vi "wash reactor.vi"(1 "channel":i8=1, 2 "Switch to position (A/B)":enum16{"A", "B"}(ring)) -> ()   [LabVIEW 2023]
panel:
  out "channel":string
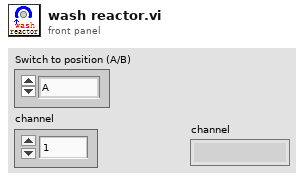
[diagram p1: front panel]
types:
  T1 = enum16{"Initialize", "Absolute Position", "Relative Pickup", "Relative Dispense", "Swich valve", "Bypass"}
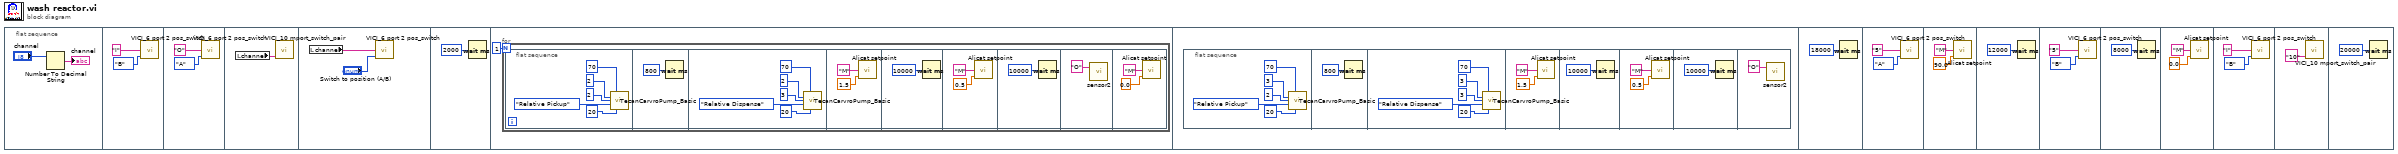
[diagram p0: block diagram]
diagram:
  n1 = flat-sequence {
    frame #0 {
      n2 = Number To Decimal String(number="channel") -> (decimal integer string=→"channel":string)  [unwired: 1 in]
    }
    frame #1 {
      n3 = call "VICI_6 port 2 pos_switch.vi"("Switch to position (A/B)"=enum16{"A", "B"}."B", "Valve ID"="I") -> ()  [unwired: 2 in, 1 out]
    }
    frame #2 {
      n4 = call "VICI_6 port 2 pos_switch.vi"("Switch to position (A/B)"=enum16{"A", "B"}."A", "Valve ID"="O") -> ()  [unwired: 2 in, 1 out]
    }
    frame #3 {
      n5 = local read "channel"() -> (w7:string)
      n6 = call "VICI_10 mport_switch_pair.vi"("Go to position"=w7) -> ()  [unwired: 3 in, 1 out]
    }
    frame #4 {
      n7 = local read "channel"() -> (w9:string)
      n8 = call "VICI_6 port 2 pos_switch.vi"("Switch to position (A/B)"="Switch to position (A/B)", "Valve ID"=w9) -> ()  [unwired: 2 in, 1 out]
    }
    frame #5 {
      n9 = Wait (ms)(milliseconds to wait=u32 2000) -> ()  [unwired: 1 out]
    }
    frame #6 {
      n10 = for {
        N: 1 -> [_]
        n11 = flat-sequence {
          frame #0 {
            n12 = call "TecanCarvroPump_Basic.vi"("Volume (μL)"=u16 70, "TecanPump address"=u8 2, "Valve"=u8 2, "Mode"=T1."Relative Pickup", "Speed (μL/s)"=u16 20) -> ()  [unwired: 10 in, 1 out]
          }
          frame #1 {
            n13 = Wait (ms)(milliseconds to wait=u32 800) -> ()  [unwired: 1 out]
          }
          frame #2 {
            n14 = call "TecanCarvroPump_Basic.vi"("Volume (μL)"=u16 70, "TecanPump address"=u8 2, "Valve"=u8 3, "Mode"=T1."Relative Dispense", "Speed (μL/s)"=u16 20) -> ()  [unwired: 10 in, 1 out]
          }
          frame #3 {
            n15 = call "Alicat setpoint.vi"("Setpoint"=1.5, "Unit ID"="M") -> ()  [unwired: 3 in]
          }
          frame #4 {
            n16 = Wait (ms)(milliseconds to wait=u32 10000) -> ()  [unwired: 1 out]
          }
          frame #5 {
            n17 = call "Alicat setpoint.vi"("Setpoint"=0.5, "Unit ID"="M") -> ()  [unwired: 3 in]
          }
          frame #6 {
            n18 = Wait (ms)(milliseconds to wait=u32 10000) -> ()  [unwired: 1 out]
          }
          frame #7 {
            n19 = call "sensor2.vi"("Sensor"="O") -> ()  [unwired: 1 in, 2 out]
          }
          frame #8 {
            n20 = call "Alicat setpoint.vi"("Setpoint"=0.0, "Unit ID"="M") -> ()  [unwired: 3 in]
          }
        }
      }
    }
    frame #7 {
      n21 = flat-sequence {
        frame #0 {
          n22 = call "TecanCarvroPump_Basic.vi"("Volume (μL)"=u16 70, "TecanPump address"=u8 3, "Valve"=u8 2, "Mode"=T1."Relative Pickup", "Speed (μL/s)"=u16 20) -> ()  [unwired: 10 in, 1 out]
        }
        frame #1 {
          n23 = Wait (ms)(milliseconds to wait=u32 800) -> ()  [unwired: 1 out]
        }
        frame #2 {
          n24 = call "TecanCarvroPump_Basic.vi"("Volume (μL)"=u16 70, "TecanPump address"=u8 3, "Valve"=u8 3, "Mode"=T1."Relative Dispense", "Speed (μL/s)"=u16 20) -> ()  [unwired: 10 in, 1 out]
        }
        frame #3 {
          n25 = call "Alicat setpoint.vi"("Setpoint"=1.5, "Unit ID"="M") -> ()  [unwired: 3 in]
        }
        frame #4 {
          n26 = Wait (ms)(milliseconds to wait=u32 10000) -> ()  [unwired: 1 out]
        }
        frame #5 {
          n27 = call "Alicat setpoint.vi"("Setpoint"=0.5, "Unit ID"="M") -> ()  [unwired: 3 in]
        }
        frame #6 {
          n28 = Wait (ms)(milliseconds to wait=u32 10000) -> ()  [unwired: 1 out]
        }
        frame #7 {
          n29 = call "sensor2.vi"("Sensor"="O") -> ()  [unwired: 1 in, 2 out]
        }
      }
    }
    frame #8 {
      n30 = Wait (ms)(milliseconds to wait=u32 18000) -> ()  [unwired: 1 out]
    }
    frame #9 {
      n31 = call "VICI_6 port 2 pos_switch.vi"("Switch to position (A/B)"=enum16{"A", "B"}."A", "Valve ID"="5") -> ()  [unwired: 2 in, 1 out]
    }
    frame #10 {
      n32 = call "Alicat setpoint.vi"("Setpoint"=90.0, "Unit ID"="M") -> ()  [unwired: 3 in]
    }
    frame #11 {
      n33 = Wait (ms)(milliseconds to wait=u32 12000) -> ()  [unwired: 1 out]
    }
    frame #12 {
      n34 = call "VICI_6 port 2 pos_switch.vi"("Switch to position (A/B)"=enum16{"A", "B"}."B", "Valve ID"="5") -> ()  [unwired: 2 in, 1 out]
    }
    frame #13 {
      n35 = Wait (ms)(milliseconds to wait=u32 8000) -> ()  [unwired: 1 out]
    }
    frame #14 {
      n36 = call "Alicat setpoint.vi"("Setpoint"=0.0, "Unit ID"="M") -> ()  [unwired: 3 in]
    }
    frame #15 {
      n37 = call "VICI_6 port 2 pos_switch.vi"("Switch to position (A/B)"=enum16{"A", "B"}."B", "Valve ID"="I") -> ()  [unwired: 2 in, 1 out]
    }
    frame #16 {
      n38 = call "VICI_10 mport_switch_pair.vi"("Go to position"="10") -> ()  [unwired: 3 in, 1 out]
    }
    frame #17 {
      n39 = Wait (ms)(milliseconds to wait=u32 20000) -> ()  [unwired: 1 out]
    }
  }
